vi "l_matr_v1.vi"() -> ()   [LabVIEW 2009]
panel:
  out "Linia selectata":bool[](array[boolean])=[FALSE, FALSE, TRUE, TRUE, FALSE]
  in  "Array 3":bool[][](array[boolean])=[[FALSE, TRUE, TRUE, TRUE, FALSE], [TRUE, FALSE, FALSE, FALSE, TRUE], [FALSE, FALSE, FALSE, FALSE, TRUE], [FALSE, FALSE, TRUE, TRUE, FALSE], [FALSE, FALSE, FALSE, FALSE, TRUE], [TRUE, FALSE, FALSE, FALSE, TRUE], [FALSE, TRUE, TRUE, TRUE, FALSE]]
  in  "Linia":u8(slide)=3 scale=6.0..0.0
  in  "Iesire":bool
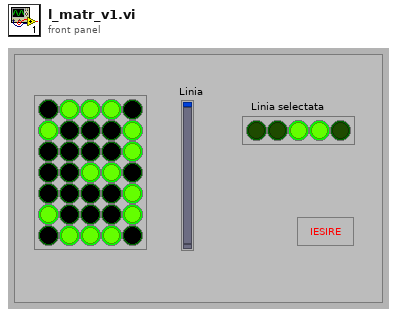
[diagram p1: front panel]
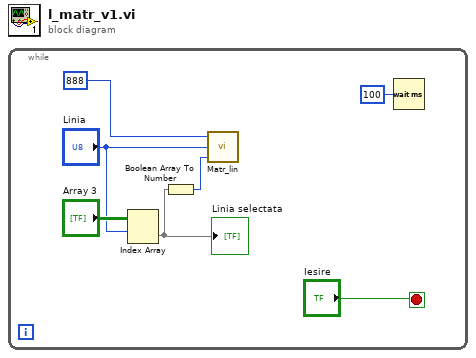
[diagram p0: block diagram]
diagram:
  n1 = while {
    stop <- "Iesire" stop-if-true
    n2 = Index Array(array="Array 3", index (row)="Linia") -> (element=w1:bool[])  [unwired: 1 in]
    "Linia selectata" <- w1
    n3 = Boolean Array To Number(Boolean array=w1) -> (number=w2:u32)
    n4 = call "Matr_lin.vi"("Date"=w2, "Linia"="Linia", "Adresa port paralel"=888) -> ()  [unwired: 2 out]
    n5 = Wait (ms)(milliseconds to wait=u32 100) -> ()  [unwired: 1 out]
  }
